vi "constants.vi"() -> ()   [LabVIEW 2013]
uses:
  <vilib>/Utility/traverseref.llb/TRef TravTarget.ctl
  <vilib>/regexp/Match Regular Expression.xnode
  <vilib>/Utility/traverseref.llb/VI Scripting - Traverse.lvlib
panel:
  out "Enum 3":enum16{"hallo2", "hallo1", "hallo"}(ring)
  out "error out":errorcluster caption="Fehler (Ausgang)"
  out "Array":string[](array[string])
  out "References":refnum<vi>[](array[refnum]) caption="Referenzen"
  out "Numerisch 2":i32
  out "Numerisch":i32
  in  "Fehler (Eingang, kein Fehler)":errorcluster
  out "String 5":string
  out "String 4":string
  out "Vor Übereinstimmung":string
  out "AlterWert":string
  in  "String 3":string
  in  "String 2":string
  out "Fehler (Ausgang)":errorcluster
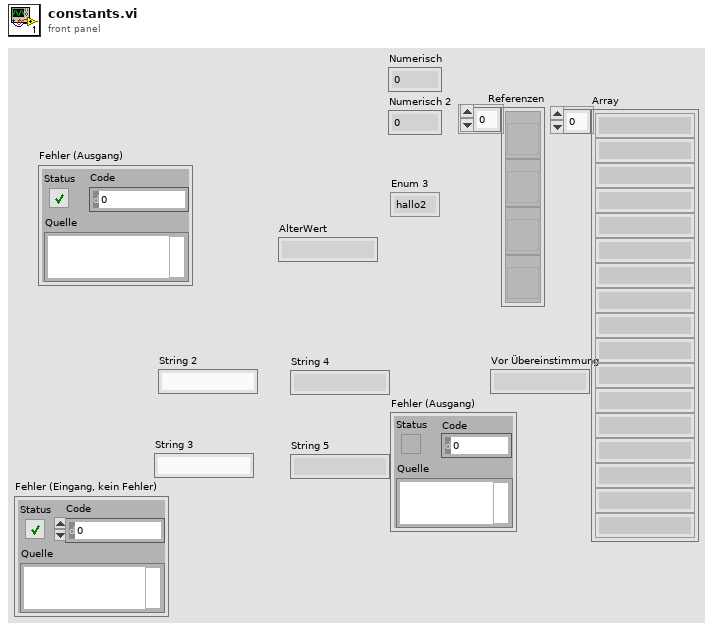
[diagram p1: front panel]
types:
  T1 = typedef "TRef TravTarget.ctl" = enum16{"FP", "BD", "Other"}
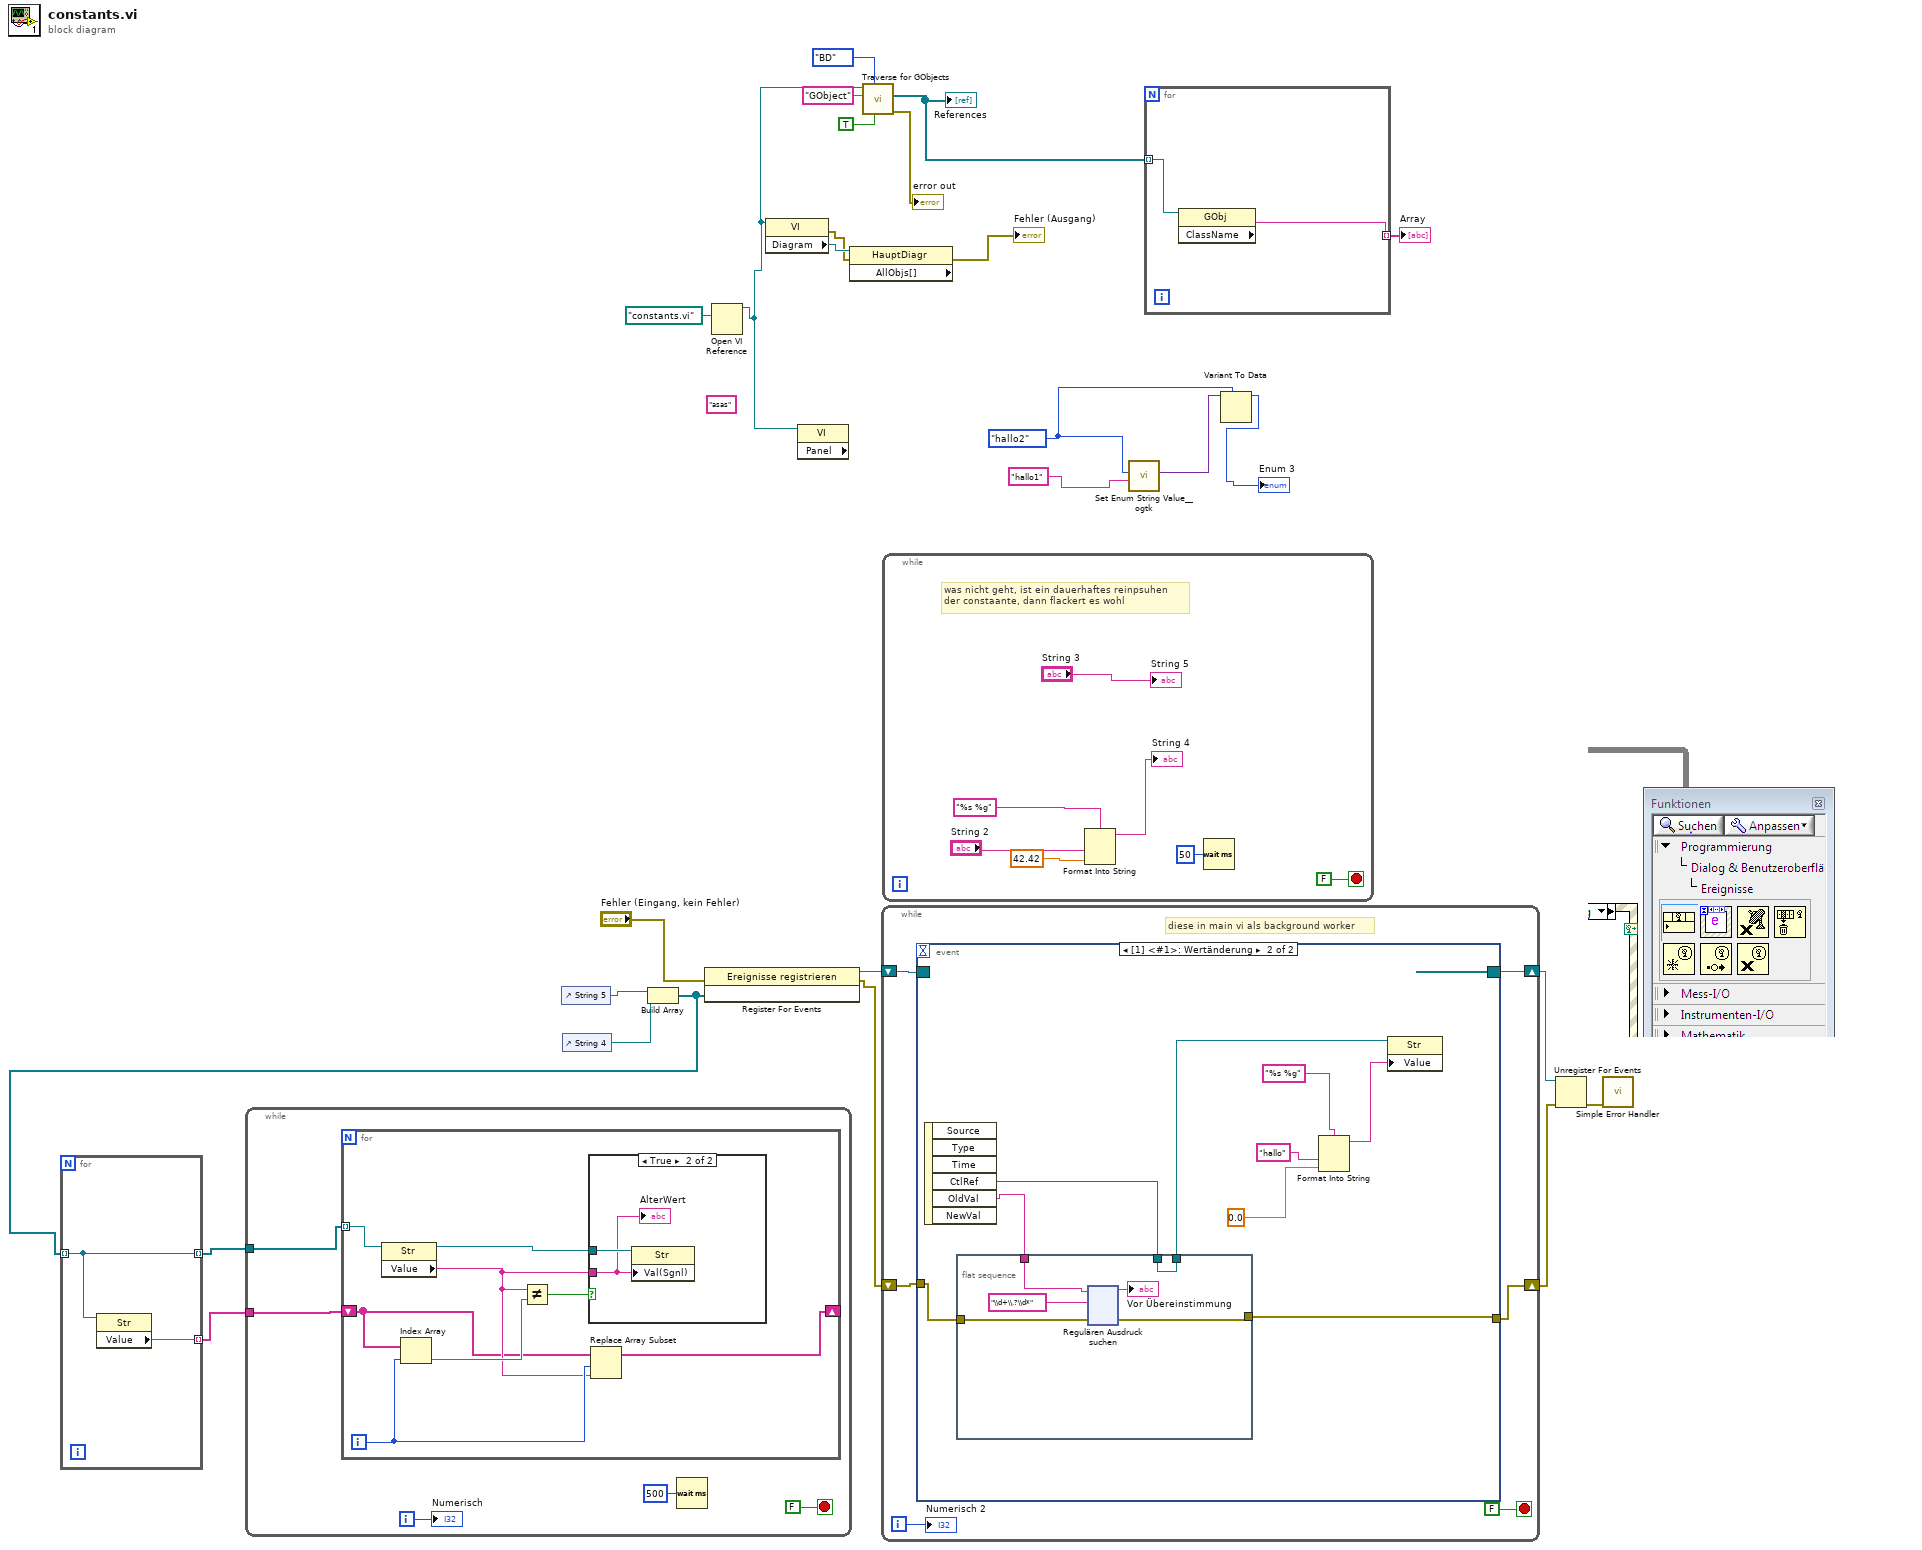
[diagram p0: block diagram]
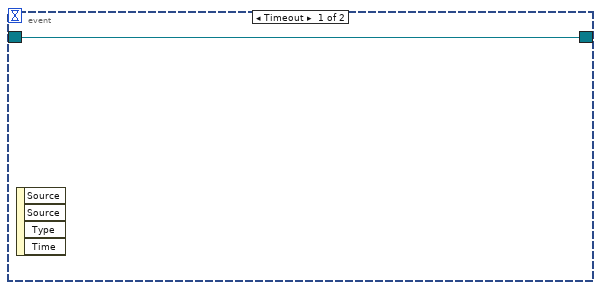
[diagram p3: hidden frame]
diagram:
  w1 = enum16{"hallo2", "hallo1", "hallo"}."hallo2" ("Enum 2")
  (unwired) "asas"
  n1 = control-ref of="String 5"() -> (w23:refnum<vi>)
  n2 = control-ref of="String 4"() -> (w22:refnum<vi>)
  n3 = Build Array(w23, w22) -> (w18:refnum<vi>[])
  n4 = for {
    tunnel: w18 -> [w28] mode=indexing
    tunnel: [w28] -> w17 mode=indexing
    tunnel: [w27] -> w16 mode=indexing
    n5 = property class="Str"(reference=w28) -> ("Value"=w27:string)  [unwired: 1 in, 2 out]
  }
  n6 = while {
    tunnel: w17 -> [w30]
    tunnel: w16 -> [w29]
    i -> [w32]
    stop <- FALSE stop-if-true
    n7 = for {
      tunnel: w30 -> [w41] mode=indexing
      shift-right: [w37] -> _
      shift-left: w29 -> [w34]
      i -> [w36]
      n8 = property class="Str"(reference=w41) -> (reference out=w40:refnum<vi>, "Value"=w35:string)  [unwired: 1 in, 1 out]
      n9 = Index Array(array=w34, index=w36) -> (element=w38:string)
      n10 = Not Equal?(x=w35, y=w38) -> (x != y?=w39:bool)
      n11 = case shown="True" w39 {
        tunnel: w40 -> [_ w43]
        tunnel: w35 -> [_ w42]
        frame False {
        }
        frame True {
          n12 = property class="Str"(reference=w43, "Val(Sgnl)"=w42) -> ()  [unwired: 1 in, 2 out]
          "AlterWert" <- w42
        }
      }
      n13 = Replace Array Subset(array=w34, new element=w35, index=w36) -> (w37:string[])
    }
    n14 = Wait (ms)(milliseconds to wait=u32 500 ("Zu wartende ms")) -> ()  [unwired: 1 out]
    "Numerisch" <- w32
  }
  n15 = register-events(error in="Fehler (Eingang, kein Fehler)", w18) -> (reference out=w26:refnum<event-registration>, error out=w20:errorcluster)  [unwired: 1 in]
  n16 = Open VI Reference(vi path=path "constants.vi" ("VI-Pfad")) -> (vi reference=w11:refnum<vi>)  [unwired: 5 in, 1 out]
  n17 = property class="VI"(reference=w11) -> (error out=w14:errorcluster, "Diagram"=w15:refnum<vi>)  [unwired: 1 in, 1 out]
  n18 = property class="VI" props=["Panel"](reference=w11) -> ()  [unwired: 1 in, 3 out]
  n19 = property class="HauptDiagr" props=["AllObjs[]"](reference=w15, error in=w14) -> (error out=→"Fehler (Ausgang)":errorcluster)  [unwired: 2 out]
  n20 = call <vilib>:"Traverse for GObjects.vi"("Traverse Generated Code (F)"=TRUE, "Traverse Target"=TRef_TravTarget."BD", "Class Name"="GObject", "VI Refnum"=w11) -> ("error out"=→"error out":errorcluster, "References"=w8:refnum<vi>[])  [unwired: 4 in, 2 out]
  "References" <- w8
  n21 = while {
    shift-right: [w47] -> w24
    shift-left: w26 -> [w48]
    shift-right: [w45] -> w19
    shift-left: w20 -> [w46]
    i -> [w44]
    stop <- FALSE stop-if-true
    # "diese in main vi als background worker"
    n22 = event shown="[1] <#1>: Wertänderung" {
      selector: w48 -> [w50 _]
      dyn-events: [w50 _] -> w47
      timeout: _ -> [_ _]
      tunnel: w46 -> [_ w53]
      tunnel: [_ w52] -> w45
      event Timeout {
        n23 = event-data() -> ()  [unwired: 1 in, 4 out]
      }
      event Value Change {
        n24 = event-data() -> ("CtlRef"=w56:refnum<vi>, "OldVal"=w54:string)  [unwired: 1 in, 4 out]
        n25 = flat-sequence {
          tunnel: w56 -> [w64]
          tunnel: [w64] -> w55
          tunnel: w54 -> [w63]
          tunnel: w53 -> [w61]
          tunnel: [w60] -> w52
          frame #0 {
            n26 = xnode "Regulären Ausdruck suchen"("Eingangs-String"=w63, "Regulärer Ausdruck"="\\d+\\.?\\d*", "Fehler (Eingang)"=w61) -> ("Vor Übereinstimmung"=→"Vor Übereinstimmung":string, "Fehler (Ausgang)"=w60:errorcluster)  [unwired: 3 in, 3 out]
          }
        }
        n27 = Format Into String(format string="%s %g" ("Wert"), "hallo" ("Eingang 1"), 0.0 ("Eingang 2")) -> (resulting string=w57:string)  [unwired: 2 in, 1 out]
        n28 = property class="Str"(reference=w55, "Value"=w57) -> ()  [unwired: 1 in, 2 out]
      }
    }
    "Numerisch 2" <- w44
  }
  n29 = while {
    stop <- FALSE stop-if-true
    # "was nicht geht, ist ein dauerhaftes reinpsuhen \nder constaante, dann flackert es wohl"
    n30 = Format Into String(format string="%s %g" ("Wert"), "String 2", 42.42 ("Eingang 2")) -> (resulting string=→"String 4":string)  [unwired: 2 in, 1 out]
    n31 = Wait (ms)(milliseconds to wait=u32 50 ("Zu wartende ms")) -> ()  [unwired: 1 out]
    "String 5" <- "String 3"
  }
  n32 = call <userlib>:"Set Enum String Value__ogtk.vi"("String Value"="hallo1", "Default Enum Value"=w1) -> ("Enum"=w4:variant)  [unwired: 8 in, 1 out]
  n33 = for {
    tunnel: w8 -> [w188] mode=indexing
    tunnel: [w187] -> w7 mode=indexing
    n34 = property class="GObj"(reference=w188) -> ("ClassName"=w187:string)  [unwired: 1 in, 2 out]
  }
  "Array" <- w7
  n35 = Variant To Data(type=w1, Variant=w4) -> (data=→"Enum 3":enum16{"hallo2", "hallo1", "hallo"})  [unwired: 1 in, 1 out]
  n36 = Unregister For Events(event registration refnum=w24, error in=w19) -> (error out=w25:errorcluster)
  n37 = call <vilib>:"Simple Error Handler.vi"("error in (no error)"=w25) -> ()  [unwired: 4 in, 5 out]
